vi "Drift Zustandsautomat.vi"(0 "Aktion":T1, 11 "error in (no error)":errorcluster caption="Fehler (Eingang, kein Fehler)") -> (2 "Anzeige aktualisieren":bool, 4 "Aktion":T1, 6 "Status":string, 10 "Start Button aktivieren":bool, 15 "error out":errorcluster caption="Fehler (Ausgang)")   [LabVIEW 2020, in "EPA 1065.lvlib" / "Gas Analyzer Drift 1065-550.lvlib"]
uses:
  Gas Analyzer Drift 1065-550.lvlib
  Aktion Drift Zustandsautomat.ctl
  Chiller NO2 1065-376/Aktion FGV Drift Daten.ctl
  Funktionstasten/Funktionstasten.lvlib
  Funktionstasten/Funktionstasten-Aktion.ctl
  Funktionstasten/Zustaende.ctl
  Seiten/CalGas Aufschaltung/FGV CalGas Aktionen.ctl
  Seiten/CalGas Aufschaltung/CalGas Aufschaltung.lvlib
  Seiten/CalGas Aufschaltung/Auswahl Aufschaltpunkt.ctl
  PNS/Aktionen FGV Grenzwerte.ctl
  PNS/PNS.lvlib
  Sprachverwaltung/Sprachverwaltung.lvlib
  Sprachverwaltung/FGV Aktion Tabelle zerlegen.ctl
  Seiten/FT-IR/FT-IR.lvlib
  EPA 1065.lvlib
  Allgemeine VIs/Aktion Test Status.ctl
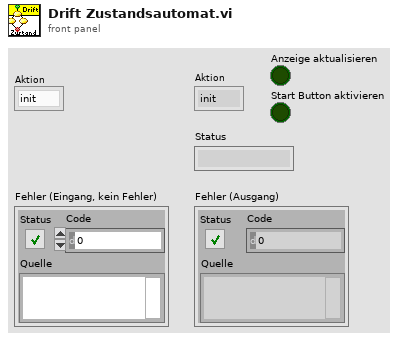
[diagram p1: front panel]
types:
  T1 = typedef "EPA 1065.lvlib/Gas Analyzer Drift 1065-550.lvlib/Aktion Drift Zustandsautomat.ctl" = enum16{"init", "lesen", "N2 aufschalten", "warten", "N2 aufzeichnen", "CG aufschalten", "CG warten", "CG aufzeichen", "Komponente Fertig", "auf nächste Komponente warten", "abbrechen", "Pre Test aktiv", "Post Test aktiv"}
  T2 = typedef "EPA 1065.lvlib/Aktion Test Status.ctl" = enum16{"init", "lesen", "prüfen", "Interference 366", "Interference 375", "Chiller läuft", "Drift läuft", "Pre Test läuft", "FID Optimization läuft", "FID Interference läuft"}
  T3 = typedef "Sprachverwaltung.lvlib/FGV Aktion Tabelle zerlegen.ctl" = enum16{"laden", "vereinzeln", "speichern"}
  T4 = typedef "CalGas Aufschaltung.lvlib/FGV CalGas Aktionen.ctl" = enum16{"lesen", "Analysator Auswahl", "Def.CalGas", "Aufschaltung CalGas", "laden", "speichern", "KAL extrahieren"}
  T5 = typedef "EPA 1065.lvlib/Gas Analyzer Drift 1065-550.lvlib/Aktion FGV Drift Daten.ctl" = enum16{"lesen", "Konfig Daten", "PDF einstellen", "laden", "speichern", "Tabelle init", "Zeile Prüfen", "Info schreiben", "Span Einstellung", "Pre Werte schreiben", "Post Werte schreiben", "NB Pre Wert schreiben", "NB Post Wert schreiben"}
  T6 = typedef "EPA 1065.lvlib/Gas Analyzer Drift 1065-550.lvlib/Aktion FGV Drift Daten.ctl" = enum16{"lesen", "Konfig Daten", "PDF einstellen", "laden", "speichern", "Tabelle init", "Info schreiben", "Pre Werte schreiben", "Zeile löschen", "Pre Werte löschen", "Post Werte löschen", "Zeile Prüfen", "Span Einstellung", "Post Werte schreiben"}
  T7 = typedef "Funktionstasten.lvlib/Funktionstasten-Aktion.ctl" = enum16{"Initialisieren", "Zustand setzen", "Taste gedrückt", "Fehler speichern", "Lesen", "Manuell", "Remote", "Bitparallel", "Samplepoint", "Zeit Prüfen", "reset Umschalten"}
  T8 = typedef "Funktionstasten.lvlib/Zustaende.ctl" = enum16{"Standby", "Pause", "Eco", "Messen", "Kalibrieren", "Spülen Filter", "Spülen Leitung", "Umgebungsluft", "0-Gas", "Cal-Gas", "CG zu PNS", "-------------", "Init 1", "Init 2", "Init 3", "Init 4", "Messen vorbereiten", "Messen durchführen", "Exit"}
  T9 = typedef "CalGas Aufschaltung.lvlib/Auswahl Aufschaltpunkt.ctl" = enum16{"über Filterblock", "Analysator direkt", "über PNS", "Entnahme"}
  T10 = typedef "PNS.lvlib/Aktionen FGV Grenzwerte.ctl" = enum16{"lesen", "Grenzw. schreiben", "Anweisungscode", "IP-Adresse", "laden", "speichern", "Anweisungscode vorgeben"}
  T11 = typedef "EPA 1065.lvlib/Gas Analyzer Drift 1065-550.lvlib/Aktion FGV Drift Daten.ctl" = enum16{"lesen", "Konfig Daten", "PDF einstellen", "laden", "speichern", "Tabelle init", "Info schreiben", "Wert schreiben", "Zeile löschen", "Pre Werte löschen", "Post Werte löschen", "Zeile Prüfen", "Span Einstellung"}
  T12 = typedef "CalGas Aufschaltung.lvlib/Aufschaltung CalGas.ctl" = cluster{"Kalibriergas":T13, "Aufschaltpunkt":T9, "Analysator":T14}
  T13 = typedef "Auswahlfeld.ctl" = u16
  T14 = typedef "CalGas Aufschaltung.lvlib/Auswahl Analysator.ctl" = enum16{"FT-IR", "FID", "PMA", "PMA/FID/FT-IR"}
  T15 = typedef "EPA 1065.lvlib/Gas Analyzer Drift 1065-550.lvlib/Konfig Daten Drift Verification.ctl" = cluster{"Bearbeiter:":string, "Pfad:":path, "Textname:":string, "CG Aufschaltzeit:":dbl, "N2 Aufschaltzeit:":dbl}
  T16 = typedef "EPA 1065.lvlib/Gas Analyzer Drift 1065-550.lvlib/Modus Drift.ctl" = u16
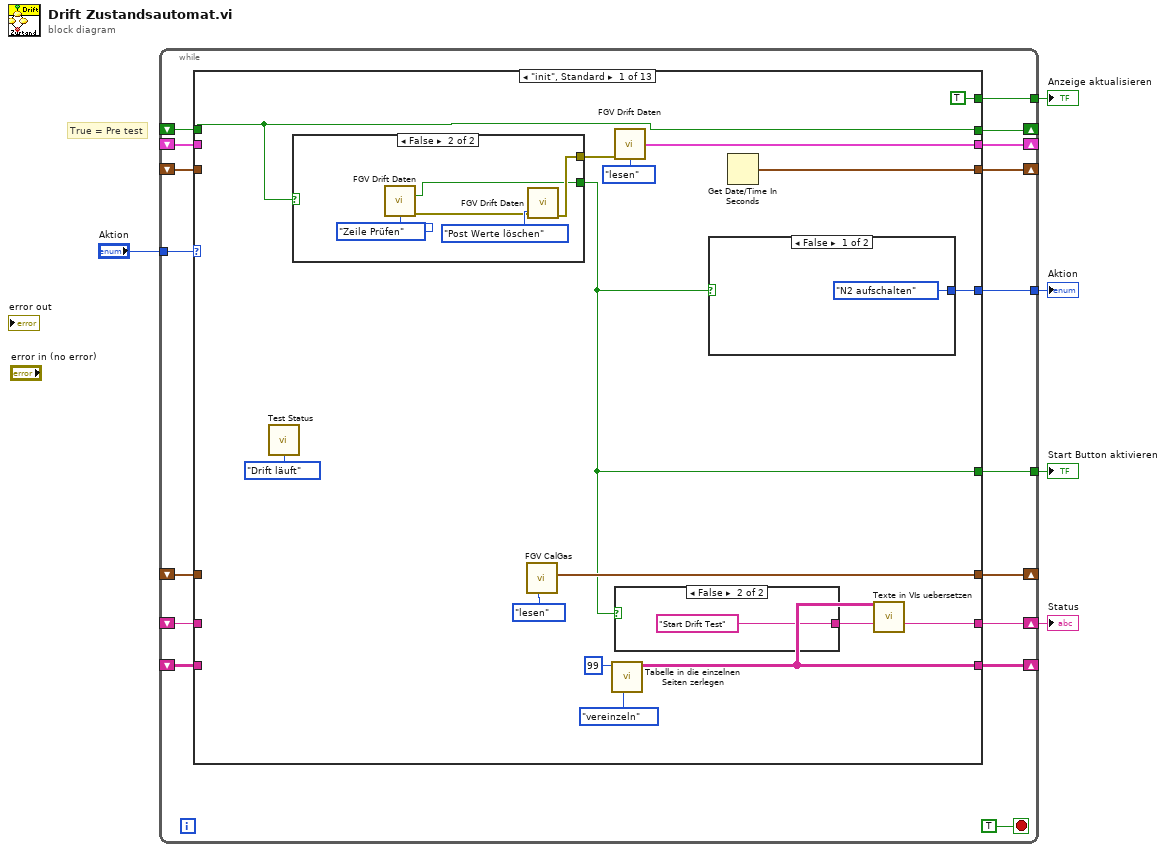
[diagram p0: block diagram]
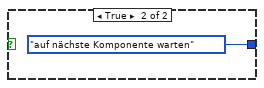
[diagram p2: hidden frame]
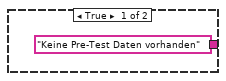
[diagram p3: hidden frame]
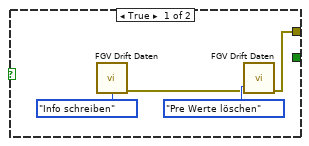
[diagram p4: hidden frame]
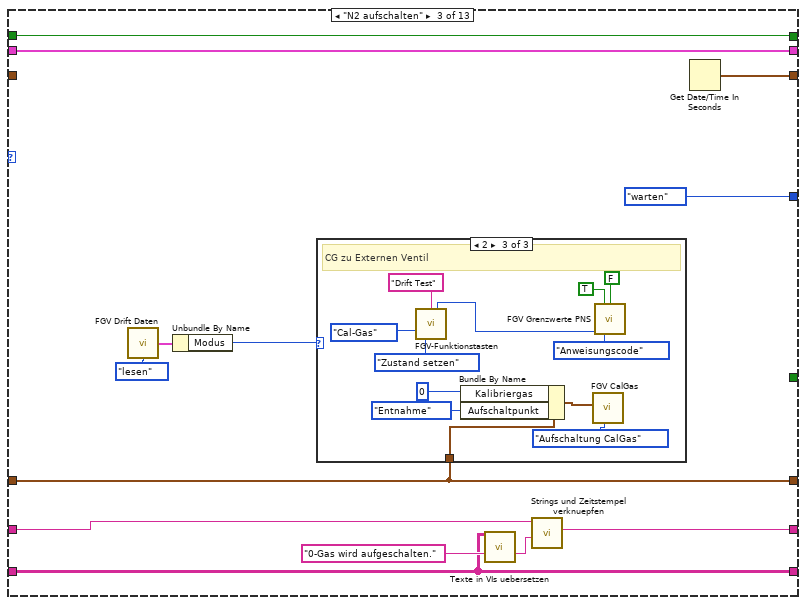
[diagram p6: hidden frame]
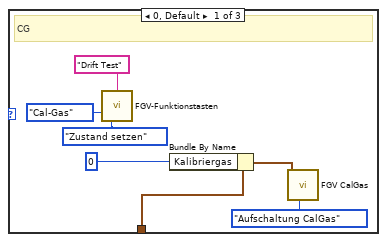
[diagram p7: hidden frame]
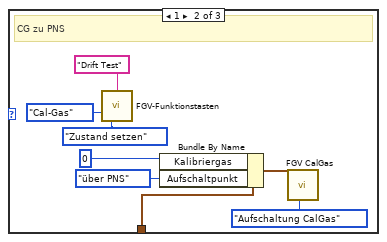
[diagram p8: hidden frame]
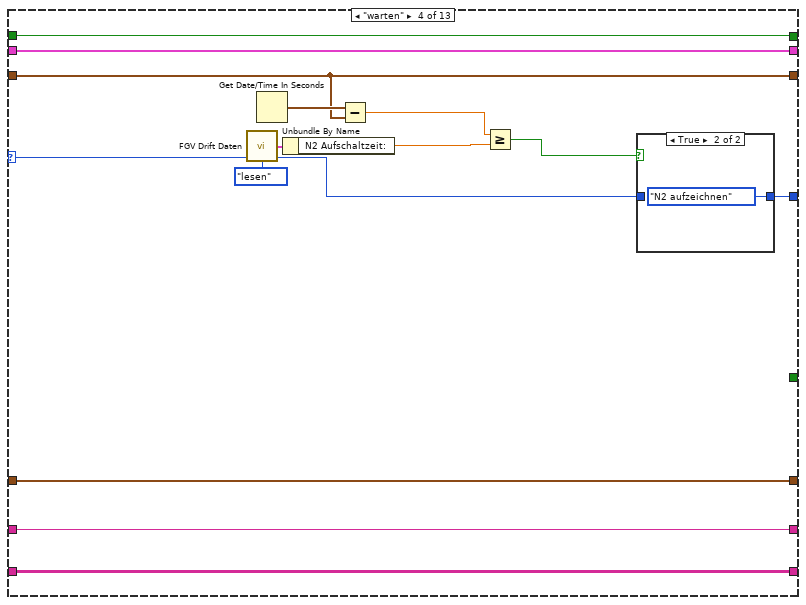
[diagram p9: hidden frame]
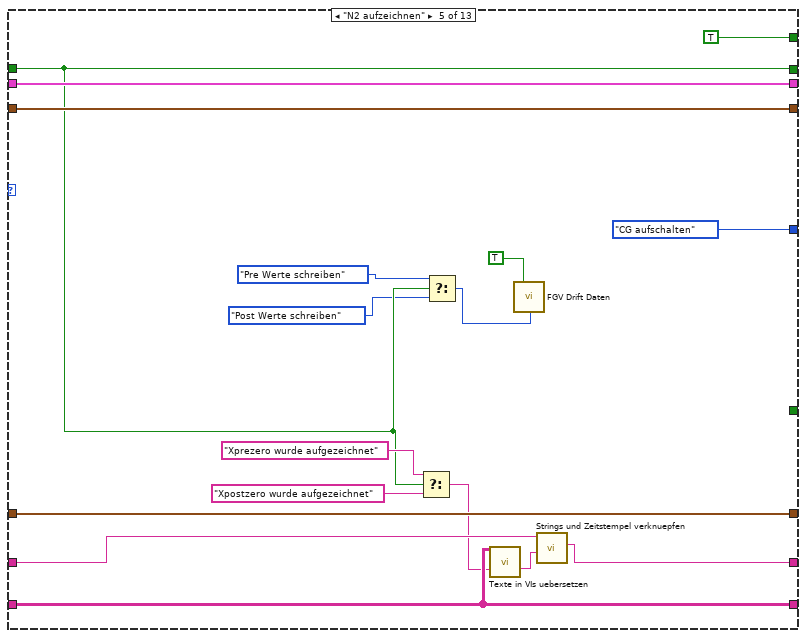
[diagram p11: hidden frame]
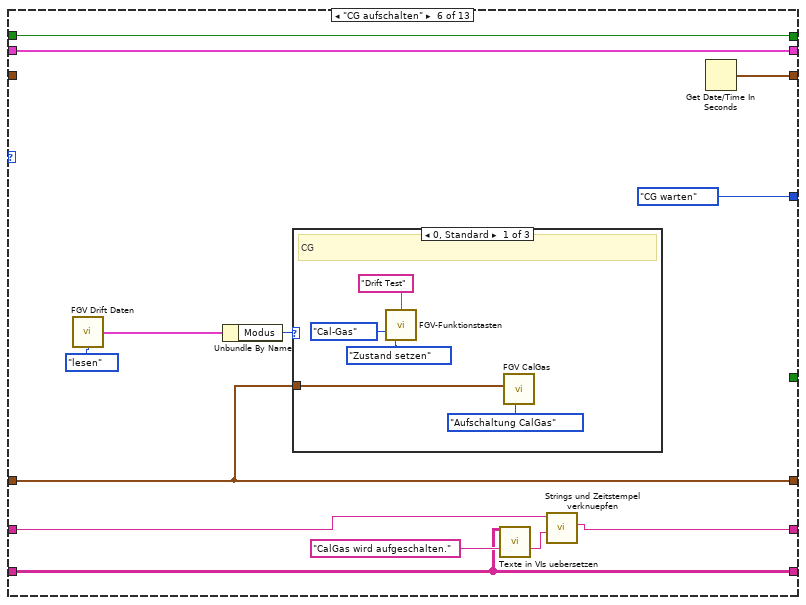
[diagram p12: hidden frame]
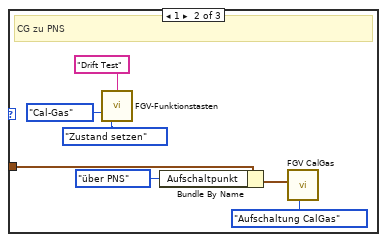
[diagram p13: hidden frame]
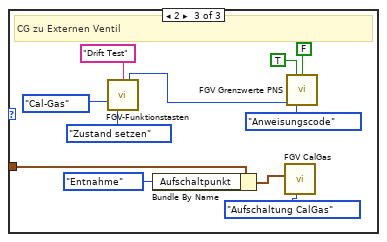
[diagram p14: hidden frame]
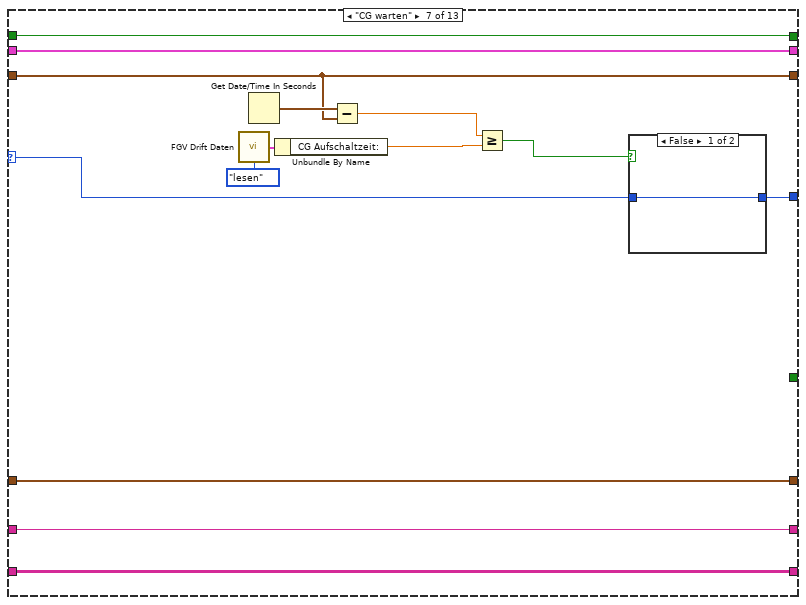
[diagram p15: hidden frame]
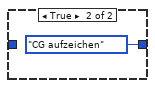
[diagram p16: hidden frame]
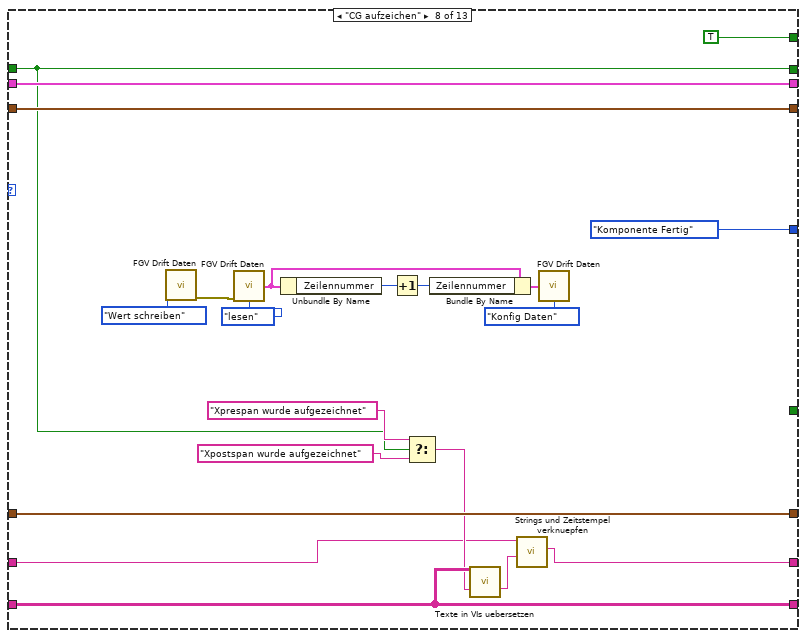
[diagram p17: hidden frame]
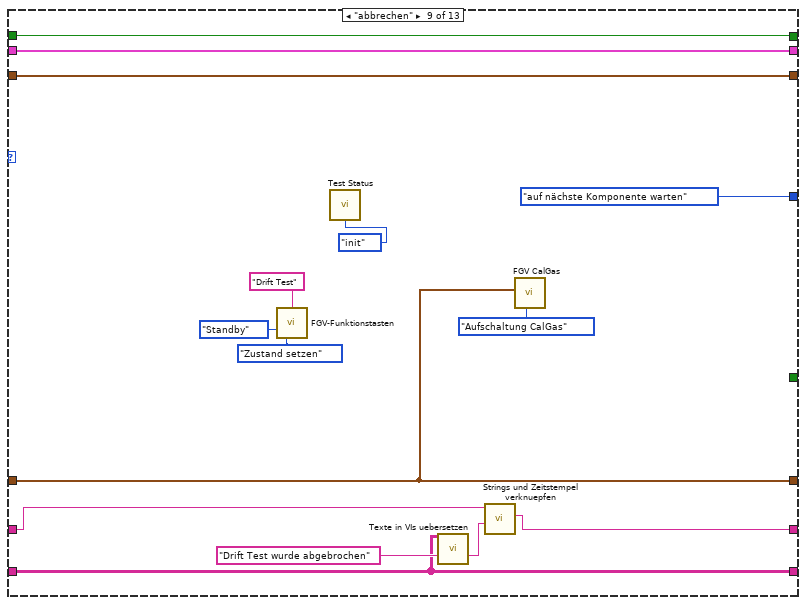
[diagram p18: hidden frame]
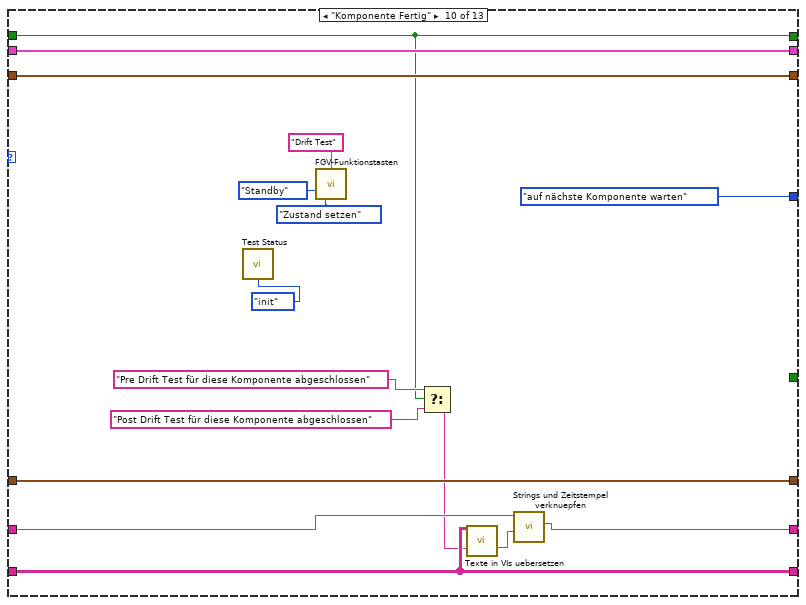
[diagram p19: hidden frame]
diagram:
  # "True = Pre test"
  n1 = while {
    tunnel: "Aktion" -> [w21]
    tunnel: [w20] -> w4
    shift-right: [w19] -> _
    shift-left: _ -> [w18]
    shift-right: [w17] -> _
    shift-left: _ -> [w16]
    shift-right: [w15] -> _
    shift-left: _ -> [w14]
    shift-right: [w13] -> _
    shift-left: _ -> [w12]
    shift-right: [w11] -> w3
    shift-left: _ -> [w10]
    shift-right: [w9] -> _
    shift-left: _ -> [w8]
    tunnel: [w7] -> w2
    tunnel: [w6] -> w1
    stop <- TRUE stop-if-true
    n2 = case shown="\"init\", Standard" w21 {
      selector: w21 -> [_ w58 _ w101 _ _ w170 _ _ _ w239 w246 w251]
      tunnel: [w38 w58 Aktion_Drift_Zustandsautomat."warten" ("Aktion") w102 Aktion_Drift_Zustandsautomat."CG aufschalten" ("Aktion") Aktion_Drift_Zustandsautomat."CG warten" ("Aktion") w171 Aktion_Drift_Zustandsautomat."Komponente Fertig" ("Aktion") Aktion_Drift_Zustandsautomat."auf nächste Komponente warten" ("Aktion") Aktion_Drift_Zustandsautomat."auf nächste Komponente warten" ("Aktion") w239 w246 w251] -> w20
      tunnel: [w35 w57 w69 w112 w131 w144 w181 w204 w214 w235 w242 w249 w256] -> w19
      tunnel: w18 -> [_ w57 w69 w112 w131 w144 w181 w204 w214 w235 w242 w249 w256]
      tunnel: [w34 w56 w67 w108 w121 w139 w172 w193 w207 w225 w238 w244 w252] -> w17
      tunnel: w16 -> [_ w56 _ w108 w121 _ w172 w193 w207 w225 w238 w244 w252]
      tunnel: [w33 w55 w66 w111 w126 w140 w180 w203 w219 w234 w241 w248 w255] -> w15
      tunnel: w14 -> [_ w55 w66 w111 w126 w140 w180 w203 w219 w234 w241 w248 w255]
      tunnel: [w30 w54 w62 w110 w129 w135 w179 w202 w208 w230 w240 w247 w254] -> w13
      tunnel: w12 -> [_ w54 w62 w110 w129 w135 w179 w202 w208 w230 w240 w247 w254]
      tunnel: [w29 w53 w60 w100 w127 w133 w169 w196 w211 w231 w237 w245 w250] -> w11
      tunnel: w10 -> [_ w53 w61 w100 w128 w134 w169 w197 w212 w232 w237 w245 w250]
      tunnel: [w27 w52 w59 w99 w119 w132 w168 w192 w206 w224 w236 TRUE FALSE] -> w9
      tunnel: w8 -> [w27 w52 w59 w99 w119 w132 w168 w192 w206 w224 w236 _ _]
      tunnel: [TRUE _ _ _ TRUE _ _ TRUE _ _ _ _ _] -> w7
      tunnel: [w25 _ _ _ _ _ _ _ _ _ _ _ _] -> w6
      frame "init", Default {
        n3 = call "Test Status.vi"("Aktion"=Aktion_Test_Status."Drift läuft") -> ()  [unwired: 11 in, 4 out]
        n4 = case shown="False" w27 {
          tunnel: [w45 w50] -> w26
          tunnel: [_ w47] -> w25
          frame True {
            n5 = call "FGV Drift Daten.vi"("Aktion"=Aktion_FGV_Drift_Daten."Info schreiben") -> ("error out"=w44:errorcluster)  [unwired: 8 in, 6 out]
            n6 = call "FGV Drift Daten.vi"("error in (no error)"=w44, "Aktion"=Aktion_FGV_Drift_Daten."Pre Werte löschen") -> ("error out"=w45:errorcluster)  [unwired: 7 in, 6 out]
          }
          frame False {
            n7 = call "FGV Drift Daten.vi"("Aktion"=Aktion_FGV_Drift_Daten."Zeile Prüfen") -> ("keine Pre Daten vorhanden"=w47:bool, "error out"=w48:errorcluster)  [unwired: 8 in, 5 out]
            n8 = call "FGV Drift Daten.vi"("error in (no error)"=w48, "Aktion"=Aktion_FGV_Drift_Daten."Post Werte löschen") -> ("error out"=w50:errorcluster)  [unwired: 7 in, 6 out]
          }
        }
        n9 = call "FGV CalGas.vi"("Aktionen"=FGV_CalGas_Aktionen."lesen") -> ("Aufschaltung CalGas"=w35:T12)  [unwired: 6 in, 4 out]
        n10 = call "Tabelle in die einzelnen Seiten zerlegen.vi"("Aktion"=FGV_Aktion_Tabelle_zerlegen."vereinzeln", "Index (Seite)"=99) -> ("Sprachliste"=w30:string[][])  [unwired: 7 in, 2 out]
        n11 = call "FGV Drift Daten.vi"("error in (no error)"=w26, "Aktion"=Aktion_FGV_Drift_Daten."lesen") -> ("Drift Konfig Daten"=w33:T15)  [unwired: 7 in, 6 out]
        n12 = case shown="False" w25 {
          tunnel: ["Keine Pre-Test Daten vorhanden" "Start Drift Test"] -> w31
          frame True {
          }
          frame False {
          }
        }
        n13 = case shown="False" w25 {
          tunnel: [Aktion_Drift_Zustandsautomat."N2 aufschalten" ("Aktion") Aktion_Drift_Zustandsautomat."auf nächste Komponente warten" ("Aktion")] -> w38
          frame False {
          }
          frame True {
          }
        }
        n14 = Get Date/Time In Seconds() -> (seconds since 1Jan1904=w34:timestamp)
        n15 = call "Texte in VIs uebersetzen.vi"("Sprachliste"=w30, "String zum Übersetzen"=w31) -> ("String zum Übersetzen"=w29:string)  [unwired: 9 in, 4 out]
      }
      frame "lesen" {
      }
      frame "N2 aufschalten" {
        n16 = call "FGV Drift Daten.vi"("Aktion"=Aktion_FGV_Drift_Daten."lesen") -> ("Drift Konfig Daten"=w68:T15)  [unwired: 8 in, 6 out]
        n17 = Unbundle By Name(w68) -> ("Modus"=w70:T16)
        n18 = case shown="2" w70 {
          tunnel: w69 -> [w73 w80 w88]
          frame 0, Default {
            # "CG"
            n19 = call "FGV-Funktionstasten.vi"("Herkunft"="Drift Test", "Zustand"=Zustaende."Cal-Gas", "Aktion"=Funktionstasten-Aktion."Zustand setzen") -> ()  [unwired: 5 in, 8 out]
            n20 = Bundle By Name(cluster=w73, "Kalibriergas"=u16 0) -> (w74:T12)
            n21 = call "FGV CalGas.vi"("Aktionen"=FGV_CalGas_Aktionen."Aufschaltung CalGas", "Aufschaltung CalGas"=w74) -> ()  [unwired: 5 in, 5 out]
          }
          frame 1 {
            # "CG zu PNS"
            n22 = call "FGV-Funktionstasten.vi"("Herkunft"="Drift Test", "Zustand"=Zustaende."Cal-Gas", "Aktion"=Funktionstasten-Aktion."Zustand setzen") -> ()  [unwired: 5 in, 8 out]
            n23 = Bundle By Name(cluster=w80, "Kalibriergas"=u16 0, "Aufschaltpunkt"=Auswahl_Aufschaltpunkt."über PNS") -> (w81:T12)
            n24 = call "FGV CalGas.vi"("Aktionen"=FGV_CalGas_Aktionen."Aufschaltung CalGas", "Aufschaltung CalGas"=w81) -> ()  [unwired: 5 in, 5 out]
          }
          frame 2 {
            # "CG zu Externen Ventil"
            n25 = call "FGV-Funktionstasten.vi"("Herkunft"="Drift Test", "Zustand"=Zustaende."Cal-Gas", "Aktion"=Funktionstasten-Aktion."Zustand setzen") -> ("Samplepoint"=w92:u16)  [unwired: 5 in, 7 out]
            n26 = Bundle By Name(cluster=w88, "Kalibriergas"=u16 0, "Aufschaltpunkt"=Auswahl_Aufschaltpunkt."Entnahme") -> (w89:T12)
            n27 = call "FGV CalGas.vi"("Aktionen"=FGV_CalGas_Aktionen."Aufschaltung CalGas", "Aufschaltung CalGas"=w89) -> ()  [unwired: 5 in, 5 out]
            n28 = call "FGV Grenzwerte PNS.vi"("T90"=TRUE ("T90 lüften"), "T90 lüften"=FALSE, "Samplepoint"=w92, "Aktionen FGV Grenzwerte"=Aktionen_FGV_Grenzwerte."Anweisungscode") -> ()  [unwired: 9 in, 3 out]
          }
        }
        n29 = call "Texte in VIs uebersetzen.vi"("Sprachliste"=w62, "String zum Übersetzen"="0-Gas wird aufgeschalten." ("String 1 hinzufügen")) -> ("String zum Übersetzen"=w63:string)  [unwired: 9 in, 4 out]
        n30 = call "Strings und Zeitstempel verknuepfen.vi"("String 1 hinzufügen"=w63, "Eingagns String"=w61) -> ("Verknüpfter String"=w60:string)  [unwired: 9 in]
        n31 = Get Date/Time In Seconds() -> (seconds since 1Jan1904=w67:timestamp)
      }
      frame "warten" {
        n32 = call "FGV Drift Daten.vi"("Aktion"=Aktion_FGV_Drift_Daten."lesen") -> ("Drift Konfig Daten"=w106:T15)  [unwired: 8 in, 6 out]
        n33 = Get Date/Time In Seconds() -> (seconds since 1Jan1904=w109:timestamp)
        n34 = Unbundle By Name(w106) -> ("N2 Aufschaltzeit:"=w105:dbl)
        n35 = Subtract(x=w109, y=w108) -> (x-y=w104:dbl)
        n36 = Greater Or Equal?(x=w104, y=w105) -> (x >= y?=w103:bool)
        n37 = case shown="True" w103 {
          tunnel: [w113 Aktion_Drift_Zustandsautomat."N2 aufzeichnen" ("Aktion")] -> w102
          tunnel: w101 -> [w113 _]
          frame False {
          }
          frame True {
          }
        }
      }
      frame "N2 aufzeichnen" {
        n38 = Select(t="Xprezero wurde aufgezeichnet" ("String 1 hinzufügen"), s=w119, f="Xpostzero wurde aufgezeichnet" ("String 1 hinzufügen")) -> (s? t:f=w124:string)
        n39 = Select(t=Aktion_FGV_Drift_Daten."Pre Werte schreiben" ("Aktion"), s=w119, f=Aktion_FGV_Drift_Daten."Post Werte schreiben" ("Aktion")) -> (s? t:f=w116:T5)
        n40 = call "Texte in VIs uebersetzen.vi"("Sprachliste"=w129, "String zum Übersetzen"=w124) -> ("String zum Übersetzen"=w130:string)  [unwired: 9 in, 4 out]
        n41 = call "FGV Drift Daten.vi"("0-Gas Wert?"=TRUE, "Aktion"=w116) -> ()  [unwired: 7 in, 7 out]
        n42 = call "Strings und Zeitstempel verknuepfen.vi"("String 1 hinzufügen"=w130, "Eingagns String"=w128) -> ("Verknüpfter String"=w127:string)  [unwired: 9 in]
      }
      frame "CG aufschalten" {
        n43 = call "FGV Drift Daten.vi"("Aktion"=Aktion_FGV_Drift_Daten."lesen") -> ("Drift Konfig Daten"=w143:T15)  [unwired: 8 in, 6 out]
        n44 = Unbundle By Name(w143) -> ("Modus"=w141:T16)
        n45 = case shown="0, Standard" w141 {
          tunnel: w144 -> [w145 w152 w159]
          frame 0, Default {
            # "CG"
            n46 = call "FGV-Funktionstasten.vi"("Herkunft"="Drift Test", "Zustand"=Zustaende."Cal-Gas", "Aktion"=Funktionstasten-Aktion."Zustand setzen") -> ()  [unwired: 5 in, 8 out]
            n47 = call "FGV CalGas.vi"("Aktionen"=FGV_CalGas_Aktionen."Aufschaltung CalGas", "Aufschaltung CalGas"=w145) -> ()  [unwired: 5 in, 5 out]
          }
          frame 1 {
            # "CG zu PNS"
            n48 = call "FGV-Funktionstasten.vi"("Herkunft"="Drift Test", "Zustand"=Zustaende."Cal-Gas", "Aktion"=Funktionstasten-Aktion."Zustand setzen") -> ()  [unwired: 5 in, 8 out]
            n49 = Bundle By Name(cluster=w152, "Aufschaltpunkt"=Auswahl_Aufschaltpunkt."über PNS") -> (w150:T12)
            n50 = call "FGV CalGas.vi"("Aktionen"=FGV_CalGas_Aktionen."Aufschaltung CalGas", "Aufschaltung CalGas"=w150) -> ()  [unwired: 5 in, 5 out]
          }
          frame 2 {
            # "CG zu Externen Ventil"
            n51 = call "FGV-Funktionstasten.vi"("Herkunft"="Drift Test", "Zustand"=Zustaende."Cal-Gas", "Aktion"=Funktionstasten-Aktion."Zustand setzen") -> ("Samplepoint"=w161:u16)  [unwired: 5 in, 7 out]
            n52 = Bundle By Name(cluster=w159, "Aufschaltpunkt"=Auswahl_Aufschaltpunkt."Entnahme") -> (w158:T12)
            n53 = call "FGV CalGas.vi"("Aktionen"=FGV_CalGas_Aktionen."Aufschaltung CalGas", "Aufschaltung CalGas"=w158) -> ()  [unwired: 5 in, 5 out]
            n54 = call "FGV Grenzwerte PNS.vi"("T90"=TRUE ("T90 lüften"), "T90 lüften"=FALSE, "Samplepoint"=w161, "Aktionen FGV Grenzwerte"=Aktionen_FGV_Grenzwerte."Anweisungscode") -> ()  [unwired: 9 in, 3 out]
          }
        }
        n55 = call "Texte in VIs uebersetzen.vi"("Sprachliste"=w135, "String zum Übersetzen"="CalGas wird aufgeschalten." ("String 1 hinzufügen")) -> ("String zum Übersetzen"=w136:string)  [unwired: 9 in, 4 out]
        n56 = call "Strings und Zeitstempel verknuepfen.vi"("String 1 hinzufügen"=w136, "Eingagns String"=w134) -> ("Verknüpfter String"=w133:string)  [unwired: 9 in]
        n57 = Get Date/Time In Seconds() -> (seconds since 1Jan1904=w139:timestamp)
      }
      frame "CG warten" {
        n58 = call "FGV Drift Daten.vi"("Aktion"=Aktion_FGV_Drift_Daten."lesen") -> ("Drift Konfig Daten"=w176:T15)  [unwired: 8 in, 6 out]
        n59 = Get Date/Time In Seconds() -> (seconds since 1Jan1904=w178:timestamp)
        n60 = Unbundle By Name(w176) -> ("CG Aufschaltzeit:"=w175:dbl)
        n61 = Subtract(x=w178, y=w172) -> (x-y=w174:dbl)
        n62 = Greater Or Equal?(x=w174, y=w175) -> (x >= y?=w173:bool)
        n63 = case shown="False" w173 {
          tunnel: [w182 Aktion_Drift_Zustandsautomat."CG aufzeichen" ("Aktion")] -> w171
          tunnel: w170 -> [w182 _]
          frame False {
          }
          frame True {
          }
        }
      }
      frame "CG aufzeichen" {
        n64 = call "FGV Drift Daten.vi"("Aktion"=Aktion_FGV_Drift_Daten."Wert schreiben") -> ("error out"=w184:errorcluster)  [unwired: 8 in, 6 out]
        n65 = call "FGV Drift Daten.vi"("error in (no error)"=w184, "Aktion"=Aktion_FGV_Drift_Daten."lesen") -> ("Drift Konfig Daten"=w190:T15)  [unwired: 7 in, 6 out]
        n66 = Unbundle By Name(w190) -> ("Zeilennummer"=w188:u32)
        n67 = Increment(x=w188) -> (x+1=w187:u32)
        n68 = Select(t="Xprespan wurde aufgezeichnet" ("String 1 hinzufügen"), s=w192, f="Xpostspan wurde aufgezeichnet" ("String 1 hinzufügen")) -> (s? t:f=w199:string)
        n69 = Bundle By Name(cluster=w190, "Zeilennummer"=w187) -> (w189:T15)
        n70 = call "Texte in VIs uebersetzen.vi"("Sprachliste"=w202, "String zum Übersetzen"=w199) -> ("String zum Übersetzen"=w198:string)  [unwired: 9 in, 4 out]
        n71 = call "Strings und Zeitstempel verknuepfen.vi"("String 1 hinzufügen"=w198, "Eingagns String"=w197) -> ("Verknüpfter String"=w196:string)  [unwired: 9 in]
        n72 = call "FGV Drift Daten.vi"("Drift Konfig Daten"=w189, "Aktion"=Aktion_FGV_Drift_Daten."Konfig Daten") -> ()  [unwired: 7 in, 7 out]
      }
      frame "abbrechen" {
        n73 = call "FGV-Funktionstasten.vi"("Herkunft"="Drift Test", "Zustand"=Zustaende."Standby", "Aktion"=Funktionstasten-Aktion."Zustand setzen") -> ()  [unwired: 5 in, 8 out]
        n74 = call "Test Status.vi"("Aktion"=Aktion_Test_Status."init") -> ()  [unwired: 11 in, 4 out]
        n75 = call "Texte in VIs uebersetzen.vi"("Sprachliste"=w208, "String zum Übersetzen"="Drift Test wurde abgebrochen") -> ("String zum Übersetzen"=w210:string)  [unwired: 9 in, 4 out]
        n76 = call "Strings und Zeitstempel verknuepfen.vi"("String 1 hinzufügen"=w210, "Eingagns String"=w212) -> ("Verknüpfter String"=w211:string)  [unwired: 9 in]
        n77 = call "FGV CalGas.vi"("Aktionen"=FGV_CalGas_Aktionen."Aufschaltung CalGas", "Aufschaltung CalGas"=w214) -> ()  [unwired: 5 in, 5 out]
      }
      frame "Komponente Fertig" {
        n78 = call "Test Status.vi"("Aktion"=Aktion_Test_Status."init") -> ()  [unwired: 11 in, 4 out]
        n79 = call "FGV-Funktionstasten.vi"("Herkunft"="Drift Test", "Zustand"=Zustaende."Standby", "Aktion"=Funktionstasten-Aktion."Zustand setzen") -> ()  [unwired: 5 in, 8 out]
        n80 = Select(t="Pre Drift Test für diese Komponente abgeschlossen" ("String 1 hinzufügen"), s=w224, f="Post Drift Test für diese Komponente abgeschlossen" ("String 1 hinzufügen")) -> (s? t:f=w226:string)
        n81 = call "Texte in VIs uebersetzen.vi"("Sprachliste"=w230, "String zum Übersetzen"=w226) -> ("String zum Übersetzen"=w233:string)  [unwired: 9 in, 4 out]
        n82 = call "Strings und Zeitstempel verknuepfen.vi"("String 1 hinzufügen"=w233, "Eingagns String"=w232) -> ("Verknüpfter String"=w231:string)  [unwired: 9 in]
      }
      frame "auf nächste Komponente warten" {
      }
      frame "Pre Test aktiv" {
      }
      frame "Post Test aktiv" {
      }
    }
  }
  "Aktion" <- w4
  "Status" <- w3
  "Anzeige aktualisieren" <- w2
  "Start Button aktivieren" <- w1
